vi "Demo.vi"() -> ()   [LabVIEW 2018, in "Thread.lvlib"]
uses:
  Thread.lvlib
  Demo Daemon.vi
panel:
  out "Thread Names":string[](array[string])
  out "Title":string
  out "?":string
  out "?":string
  out "?":string
  out "error out":errorcluster
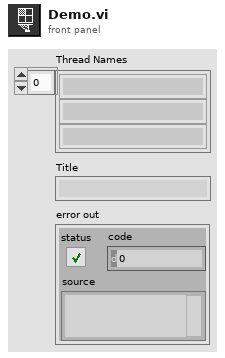
[diagram p1: front panel]
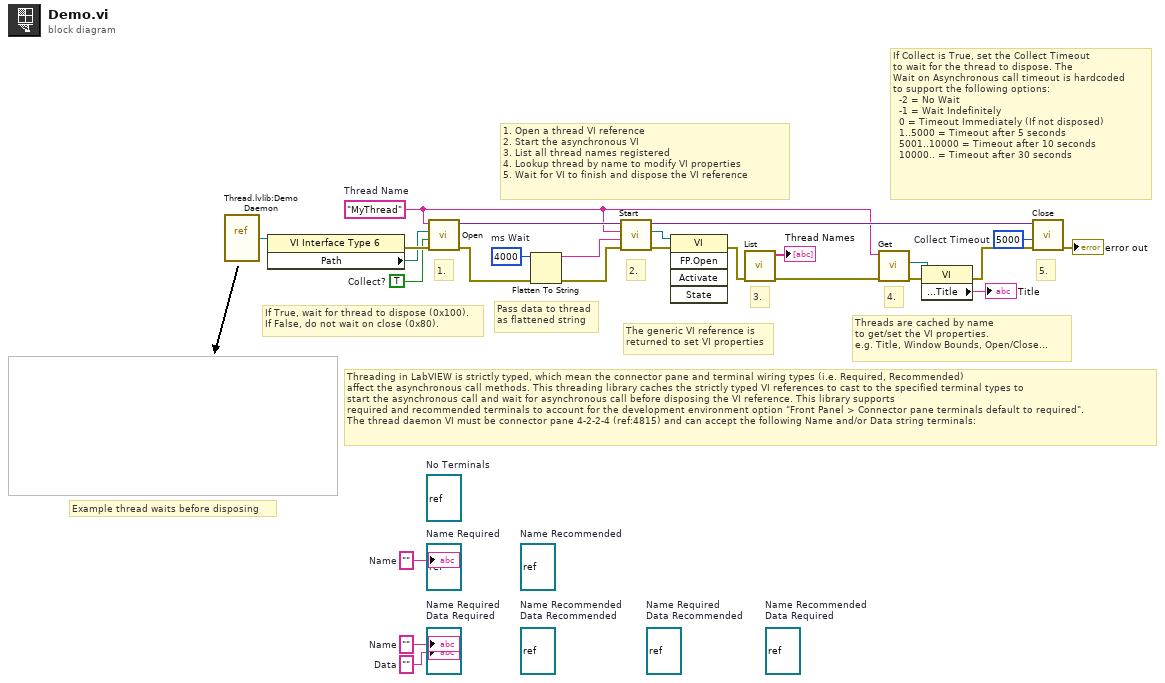
[diagram p0: block diagram]
diagram:
  w9 = ""  # Data
  w10 = ""  # Name
  w11 = ""  # Name
  (unwired) refnum<vi> refnum  # Name Recommended Data Required
  (unwired) refnum<vi> refnum  # Name Required Data Recommended
  (unwired) refnum<vi> refnum  # Name Recommended Data Recommended
  (unwired) refnum<vi> refnum  # Name Required Data Required
  (unwired) refnum<vi> refnum  # Name Recommended
  (unwired) refnum<vi> refnum  # Name Required
  (unwired) refnum<vi> refnum  # No Terminals
  w14 = 5000  # Collect Timeout
  w18 = u32 4000  # ms Wait
  w22 = TRUE  # Collect?
  w8 = "MyThread"  # Thread Name
  # "If Collect is True, set the Collect Timeout\nto wait for the thread to dispose. The\nWait on Asynchronous call timeout is hardcoded\nto support the following options:\n  -2 = No Wait\n  -1 = Wait Indefinitely\n  0 = Timeout Immediately (If not disposed)\n  1..5000 = Timeout after 5 seconds\n  5001..10000 = Timeout after 10 seconds\n  10000.. = Timeout after 30 seconds"
  # "3."
  # "Threads are cached by name\nto get/set the VI properties.\ne.g. Title, Window Bounds, Open/Close..."
  # "4."
  # "Example thread waits before disposing"
  # "If True, wait for thread to dispose (0x100).\nIf False, do not wait on close (0x80)."
  # "The generic VI reference is\nreturned to set VI properties"
  # "Threading in LabVIEW is strictly typed, which mean the connector pane and terminal wiring types (i.e. Required, Recommended)\naffect the asynchronous call methods. This threading library caches the strictly typed VI references to cast to the specified terminal types to\nstart the asynchronous call and wait for asynchronous call before disposing the VI reference. This library supports\nrequired and recommended terminals to account for the development environment option \"Front Panel > Connector pane terminals default to required\".\nThe thread daemon VI must be connector pane 4-2-2-4 (ref:4815) and can accept the following Name and/or Data string terminals:"
  # "1. Open a thread VI reference\n2. Start the asynchronous VI\n3. List all thread names registered\n4. Lookup thread by name to modify VI properties\n5. Wait for VI to finish and dispose the VI reference"
  # "5."
  # "2."
  # "1."
  # "Pass data to thread\nas flattened string"
  n1 = vi-ref "Thread.lvlib:Demo Daemon.vi"() -> (w24:refnum<vi>)
  n2 = property class="VI Interface Type 6"(reference=w24) -> (error out=w25:errorcluster, "Path"=w23:path)  [unwired: 1 in, 1 out]
  n3 = call "Open.vi"("error in (no error)"=w25, "Collect? (T)"=w22, "VI Path"=w23, "Thread Name"=w8) -> ("error out"=w20:errorcluster, "VI Reference"=w21:variant)  [unwired: 5 in, 1 out]
  n4 = Flatten To String(anything=w18, error in (no error)=w20) -> (data string=w17:string, error out=w19:errorcluster)  [unwired: 2 in, 1 out]
  n5 = call "Start.vi"("error in (no error)"=w19, "Data"=w17, "Name"=w8, "VI Reference in"=w21) -> ("error out"=w16:errorcluster, "Generic VI Reference"=w12:refnum<vi>, "VI Reference out"=w15:variant)  [unwired: 5 in]
  n6 = invoke class="VI" method="FP.Open"(reference=w12, error in=w16) -> (error out=w3:errorcluster)  [unwired: 3 in, 4 out]
  n7 = call "List.vi"("error in (no error)"=w3) -> ("error out"=w2:errorcluster, "Thread Names"=→"Thread Names":string[])  [unwired: 9 in]
  n8 = call "Get.vi"("error in (no error)"=w2, "Thread Name"=w8) -> ("error out"=w7:errorcluster, "Generic VI Reference"=w6:refnum<vi>)  [unwired: 6 in, 2 out]
  n9 = property class="VI"(reference=w6, error in=w7) -> (error out=w4:errorcluster, "Front Panel.Title"=→"Title":string)  [unwired: 1 out]
  n10 = call "Close.vi"("error in (no error)"=w4, "Collect Timeout (-2=No collect) [-2,-1,0s,5s,10s,30s]"=w14, "VI Reference in"=w15) -> ("error out"=→"error out":errorcluster)  [unwired: 8 in]
  "?" <- w11
  "?" <- w10
  "?" <- w9
